vi "ReplyNoErr.vi"() -> (0 "msg out":string)   [LabVIEW 2015]
doc: "Replies with an error code"
uses:
  MessageBuilding/std_msgs/subs/i16Scalar.vi
  MessageBuilding/std_msgs/subs/stringScalar.vi
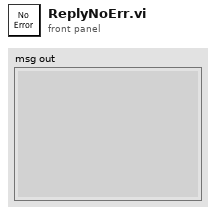
[diagram p1: front panel]
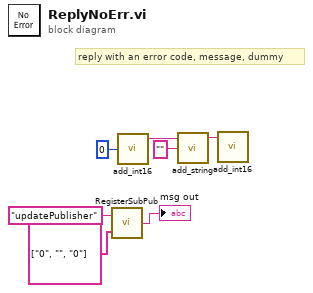
[diagram p0: block diagram]
diagram:
  # "reply with an error code, message, dummy"
  n1 = call "RegisterSubPub.vi"("Parameters"=string[] ["0", "", "0"], "MethodName"="updatePublisher") -> ("XML"=→"msg out":string)
  n2 = call-poly "add_int16.vi"("Numeric"=i16 0) -> ("msg out"=w4:string)  [unwired: 4 in]
  n3 = call-poly "add_string.vi"("String"="", "msg in"=w4) -> ("msg out"=w5:string)  [unwired: 3 in]
  n4 = call-poly "add_int16.vi"("msg in"=w5) -> ()  [unwired: 4 in, 1 out]
